vi "Configure Measurement Type.vi"(0 "VISA resource name":refnum<visa-resource-name>, 1 "Enable Clear (F: Disable)":bool, 2 "Enable Statistics Reset (F: Disable)":bool, 5 "Measurement Type (0: Peak-Peak)":i32(ring) items=["Peak-Peak", "Maximum", "Mimimum", "Amplitude", "Top", "Base", "Overshoot", "Preshoot", "Average - N Cycles", "Average - Full Screen", "DC RMS - N Cycles", "DC RMS - Full Screen", "AC RMS - N Cycles", "AC RMS - Full Screen (Std Dev)", "Ratio", "Period", "Frequency", "Counter", "+Width", "-Width", "Burst Width", "Duty Cycle", "Rise Time", "Fall Time", "Delay", "Phase", "X minY", "X maxY", "Positive Pulse Count", "Negative Pulse Count", "Raising Edge Count", "Falling Edge Count", "Area - N Cycle", "Area - Full Screen"], 7 "Measurement Source 1 (0: Channel 1)":i32(ring) items=["Channel 1"=0, "Channel 2"=1, "Channel 3"=2, "Channel 4"=3, "Math"=4, "Waveform Memory 1"=5, "Waveform Memory 2"=6, "D0"=13, "D1"=14, "D2"=15, "D3"=16, "D4"=17, "D5"=18, "D6"=19, "D7"=20, "D8"=21, "D9"=22, "D10"=23, "D11"=24, "D12"=25, "D13"=26, "D14"=27, "D15"=28, "External"=29, "Function"=32], 9 "Measurement Source 2 (1: Channel 2)":i32(ring)=1 items=["Channel 1", "Channel 2", "Channel 3", "Channel 4", "Math", "Waveform Memory 1", "Waveform Memory 2"], 11 "error in (no error)":errorcluster) -> (4 "VISA resource name out":refnum<visa-resource-name>, 15 "error out":errorcluster)   [LabVIEW 2010, in "Agilent 2000 3000 X-Series.lvlib"]
doc: "Configures the measurement type."
uses:
  <instrlib>/Agilent 2000 3000 X-Series/Agilent 2000 3000 X-Series.lvlib
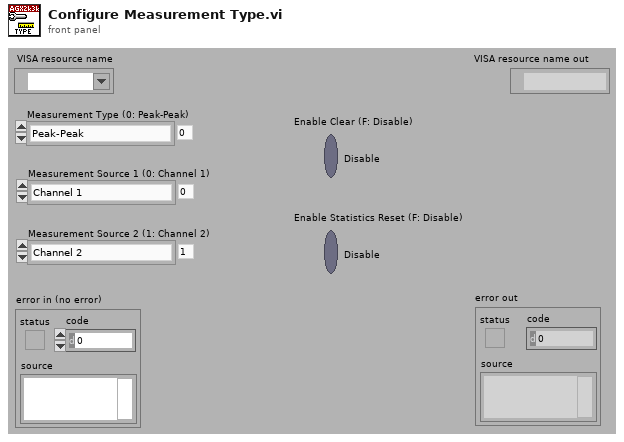
[diagram p1: front panel]
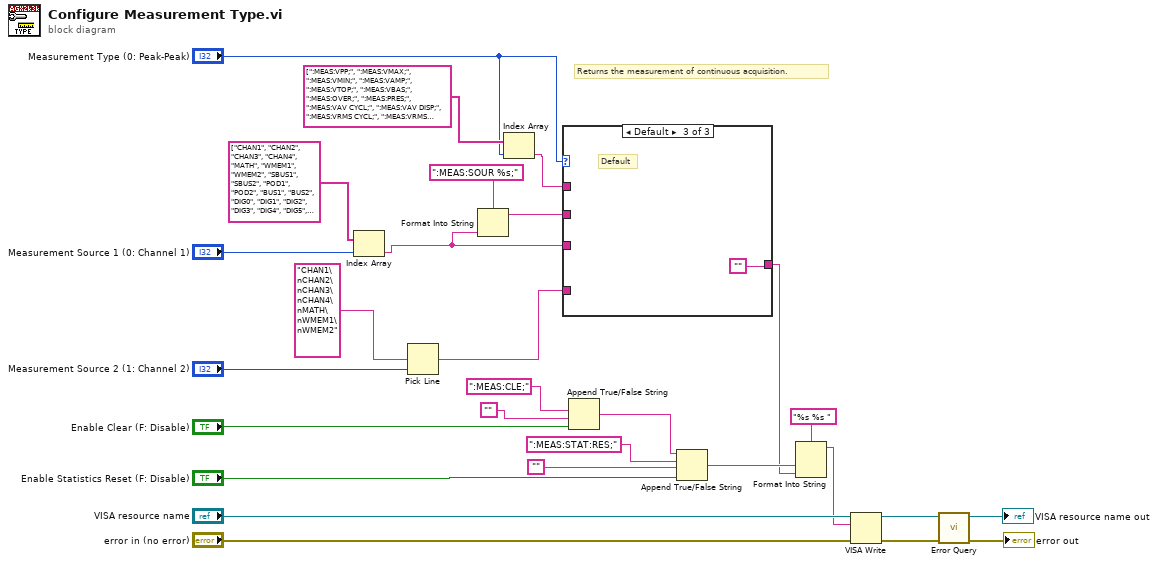
[diagram p0: block diagram]
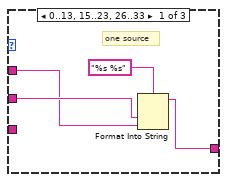
[diagram p2: hidden frame]
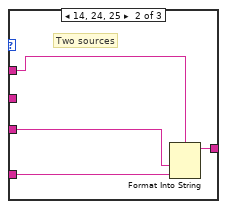
[diagram p3: hidden frame]
diagram:
  # "Returns the measurement of continuous acquisition."
  n1 = Index Array(array=string[] ["CHAN1", "CHAN2", "CHAN3", "CHAN4", "MATH", "WMEM1", "WMEM2", "SBUS1", "SBUS2", "POD1", "POD2", "BUS1", "BUS2", "DIG0", "DIG1", "DIG2", "DIG3", "DIG4", "DIG5", "DIG6", "DIG7", "DIG8", "DIG9", "DIG10", "DIG11", "DIG12", "DIG13", "DIG14", "DIG15", "EXT", "LINE", "WGEN", "FUNC"], index="Measurement Source 1 (0: Channel 1)") -> (element=w5:string)
  n2 = Pick Line(multi-line string="CHAN1\nCHAN2\nCHAN3\nCHAN4\nMATH\nWMEM1\nWMEM2", line index="Measurement Source 2 (1: Channel 2)") -> (output string=w28:string)  [unwired: 1 out]
  n3 = Format Into String(format string=":MEAS:SOUR %s;", w5) -> (resulting string=w24:string)  [unwired: 2 in, 1 out]
  n4 = Index Array(array=string[] [":MEAS:VPP;", ":MEAS:VMAX;", ":MEAS:VMIN;", ":MEAS:VAMP;", ":MEAS:VTOP;", ":MEAS:VBAS;", ":MEAS:OVER;", ":MEAS:PRES;", ":MEAS:VAV CYCL;", ":MEAS:VAV DISP;", ":MEAS:VRMS CYCL;", ":MEAS:VRMS DISP;", ":MEAS:VRMS CYCL;", ":MEAS:VRMS DISP;", ":MEAS:VRAT %s, %s;", ":MEAS:PER;", ":MEAS:FREQ;", ":MEAS:COUN;", ":MEAS:PWID;", ":MEAS:NWID;", ":MEAS:BWID;", ":MEAS:DUTY;", ":MEAS:RIS;", ":MEAS:FALL;", ":MEAS:DEL %s, %s;", ":MEAS:PHAS %s, %s;", ":MEAS:XMIN;", ":MEAS:XMAX;", ":MEAS:PPUL;", ":MEAS:NPUL;", ":MEAS:PEDG;", ":MEAS:NEDG;", ":MEAS:ARE CYCL;", ":MEAS:ARE DISP;"] ("Array"), index="Measurement Type (0: Peak-Peak)") -> (element=w4:string)
  n5 = case shown="Default" "Measurement Type (0: Peak-Peak)" {
    tunnel: w5 -> [_ w36 _]
    tunnel: w28 -> [_ w35 _]
    tunnel: [w29 w34 ""] -> w17
    tunnel: w24 -> [w31 _ _]
    tunnel: w4 -> [w30 w33 _]
    frame 0..13, 15..23, 26..33 {
      # "one source"
      n6 = Format Into String(format string="%s %s", w31, w30) -> (resulting string=w29:string)  [unwired: 2 in, 1 out]
    }
    frame 14, 24, 25 {
      # "Two sources"
      n7 = Format Into String(format string=w33, w36, w35) -> (resulting string=w34:string)  [unwired: 2 in, 1 out]
    }
    frame Default {
      # "Default"
    }
  }
  n8 = Append True/False String(1:"Enable Clear (F: Disable)", 2:"", 3:":MEAS:CLE;") -> (0:w16:string)  [unwired: 1 out]
  n9 = Append True/False String(1:"Enable Statistics Reset (F: Disable)", 2:"", 3:":MEAS:STAT:RES;", 4:w16) -> (0:w18:string)
  n10 = Format Into String(format string="%s %s ", w18, w17) -> (resulting string=w7:string)  [unwired: 2 in, 1 out]
  n11 = VISA Write(VISA resource name="VISA resource name", write buffer=w7, error in (no error)="error in (no error)") -> (VISA resource name out=w11:refnum<visa-resource-name>, error out=w10:errorcluster)  [unwired: 1 out]
  n12 = call <instrlib>:"Error Query.vi"("error in (no error)"=w10, "VISA resource name"=w11) -> ("error out"=→"error out":errorcluster, "VISA resource name out"=→"VISA resource name out":refnum<visa-resource-name>)  [unwired: 8 out]
